vi "escape json string.vi"(11 "base string":string) -> (3 "String out":string)   [LabVIEW 2013, in "json generator.lvlib"]
uses:
  json generator.lvlib
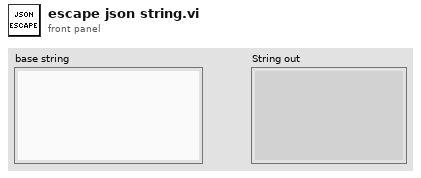
[diagram p1: front panel]
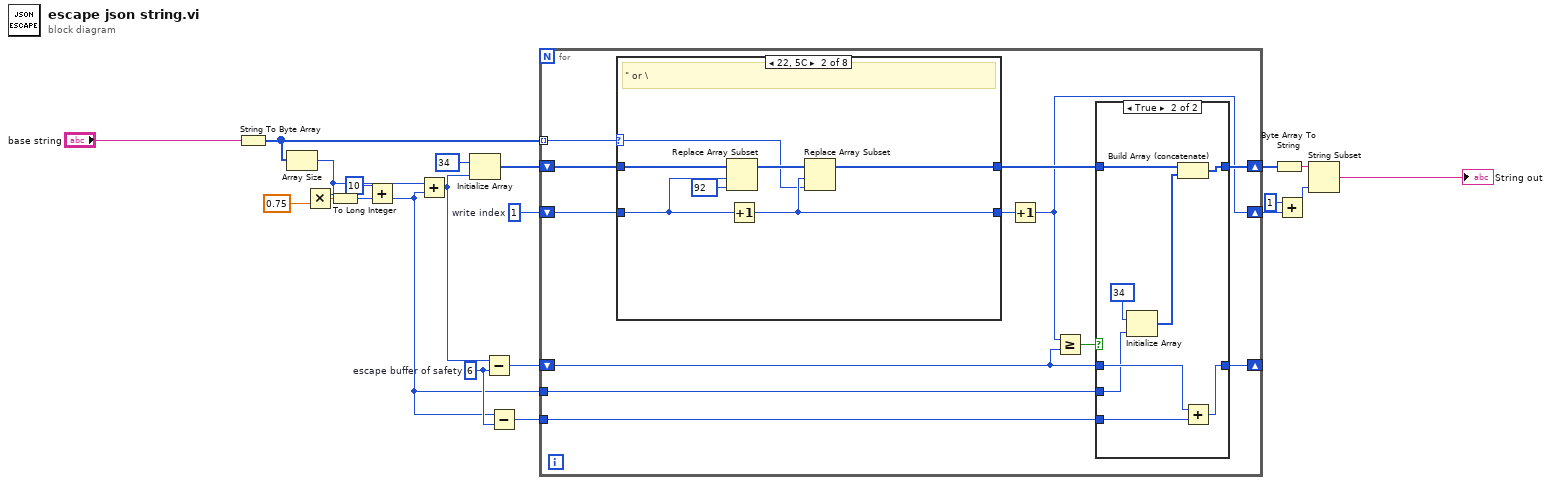
[diagram p0: block diagram]
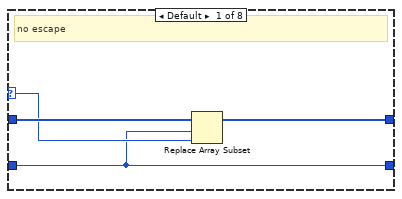
[diagram p3: hidden frame]
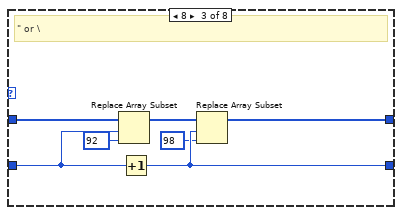
[diagram p4: hidden frame]
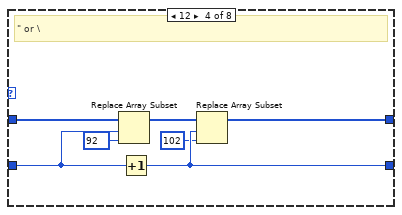
[diagram p5: hidden frame]
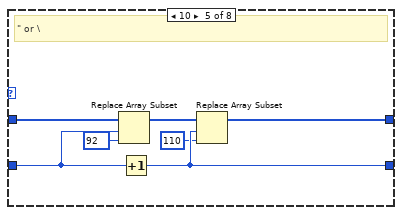
[diagram p6: hidden frame]
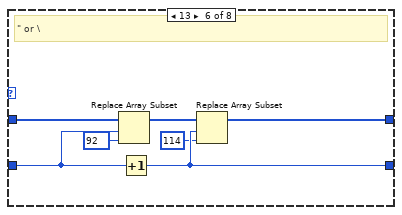
[diagram p7: hidden frame]
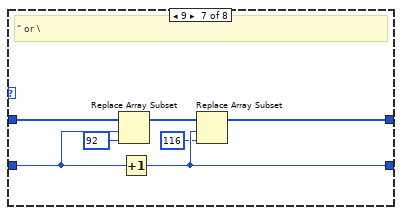
[diagram p8: hidden frame]
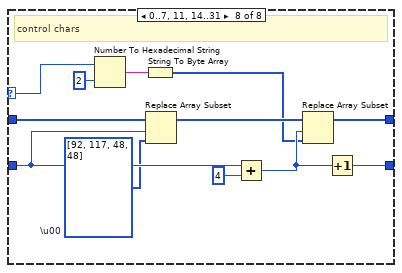
[diagram p9: hidden frame]
diagram:
  w6 = 6  # escape buffer of safety
  w18 = 1  # write index
  n1 = String To Byte Array(string="base string") -> (unsigned byte array=w12:u8[])
  n2 = Array Size(array=w12) -> (size(s)=w10:i32)
  n3 = Multiply(x=w10, y=0.75) -> (x*y=w13:dbl)
  n4 = To Long Integer(number=w13) -> (32bit integer=w7:i32)
  n5 = Add(x=10, y=w7) -> (x+y=w3:i32)
  n6 = Add(x=w10, y=w3) -> (x+y=w9:i32)
  n7 = Initialize Array(u8 34, w9) -> (w15:u8[])
  n8 = Subtract(x=w9, y=w6) -> (x-y=w8:i32)
  n9 = Subtract(x=w3, y=w6) -> (x-y=w5:i32)
  n10 = for {
    shift-right: [w30] -> w17
    shift-left: w15 -> [w33]
    shift-right: [w23] -> w11
    shift-left: w18 -> [w32]
    tunnel: w12 -> [w31] mode=indexing
    shift-right: [w27] -> _
    shift-left: w8 -> [w26]
    tunnel: w3 -> [w25]
    tunnel: w5 -> [w24]
    n11 = case shown="22, 5C" w31 {
      selector: w31 -> [w45 w49 _ _ _ _ _ w98]
      tunnel: w33 -> [w47 w54 w61 w68 w75 w82 w89 w101]
      tunnel: [w46 w51 w58 w65 w72 w79 w86 w100] -> w29
      tunnel: w32 -> [w44 w52 w59 w66 w73 w80 w87 w99]
      tunnel: [w44 w50 w57 w64 w71 w78 w85 w90] -> w28
      frame Default {
        # "no escape"
        n12 = Replace Array Subset(array=w47, new element=w45, index=w44) -> (w46:u8[])
      }
      frame 34, 92 {
        # "\" or \\"
        n13 = Replace Array Subset(array=w54, new element=u8 92 ("new element/subarray"), index=w52) -> (w53:u8[])
        n14 = Increment(x=w52) -> (x+1=w50:i32)
        n15 = Replace Array Subset(array=w53, new element=w49, index=w50) -> (w51:u8[])
      }
      frame 8 {
        # "\" or \\"
        n16 = Replace Array Subset(array=w61, new element=u8 92 ("new element/subarray"), index=w59) -> (w60:u8[])
        n17 = Increment(x=w59) -> (x+1=w57:i32)
        n18 = Replace Array Subset(array=w60, new element=u8 98 ("new element/subarray"), index=w57) -> (w58:u8[])
      }
      frame 12 {
        # "\" or \\"
        n19 = Replace Array Subset(array=w68, new element=u8 92 ("new element/subarray"), index=w66) -> (w67:u8[])
        n20 = Increment(x=w66) -> (x+1=w64:i32)
        n21 = Replace Array Subset(array=w67, new element=u8 102 ("new element/subarray"), index=w64) -> (w65:u8[])
      }
      frame 10 {
        # "\" or \\"
        n22 = Replace Array Subset(array=w75, new element=u8 92 ("new element/subarray"), index=w73) -> (w74:u8[])
        n23 = Increment(x=w73) -> (x+1=w71:i32)
        n24 = Replace Array Subset(array=w74, new element=u8 110 ("new element/subarray"), index=w71) -> (w72:u8[])
      }
      frame 13 {
        # "\" or \\"
        n25 = Replace Array Subset(array=w82, new element=u8 92 ("new element/subarray"), index=w80) -> (w81:u8[])
        n26 = Increment(x=w80) -> (x+1=w78:i32)
        n27 = Replace Array Subset(array=w81, new element=u8 114 ("new element/subarray"), index=w78) -> (w79:u8[])
      }
      frame 9 {
        # "\" or \\"
        n28 = Replace Array Subset(array=w89, new element=u8 92 ("new element/subarray"), index=w87) -> (w88:u8[])
        n29 = Increment(x=w87) -> (x+1=w85:i32)
        n30 = Replace Array Subset(array=w88, new element=u8 116 ("new element/subarray"), index=w85) -> (w86:u8[])
      }
      frame 0..7, 11, 14..31 {
        w91 = u8[] [92, 117, 48, 48]  # \u00
        # "control chars"
        n31 = Number To Hexadecimal String(1:i16 2 ("width (-)"), 2:w98) -> (0:w93:string)
        n32 = String To Byte Array(string=w93) -> (unsigned byte array=w95:u8[])
        n33 = Replace Array Subset(array=w101, new element=w91, index=w99) -> (w97:u8[])
        n34 = Add(x=w99, y=4) -> (x+y=w96:i32)
        n35 = Replace Array Subset(array=w97, new element=w95, index=w96) -> (w100:u8[])
        n36 = Increment(x=w96) -> (x+1=w90:i32)
      }
    }
    n37 = Increment(x=w28) -> (x+1=w23:i32)
    n38 = Greater Or Equal?(x=w23, y=w26) -> (x >= y?=w22:bool)
    n39 = case shown="True" w22 {
      tunnel: [w35 w38] -> w30
      tunnel: w29 -> [w35 w39]
      tunnel: [w34 w41] -> w27
      tunnel: w26 -> [w34 w42]
      tunnel: w25 -> [_ w40]
      tunnel: w24 -> [_ w43]
      frame False {
      }
      frame True {
        n40 = Initialize Array(u8 34, w40) -> (w37:u8[])
        n41 = Build Array (concatenate)(w39, w37) -> (w38:u8[])
        n42 = Add(x=w42, y=w43) -> (x+y=w41:i32)
      }
    }
  }
  n43 = Byte Array To String(unsigned byte array=w17) -> (string=w19:string)
  n44 = Add(x=1, y=w11) -> (x+y=w4:i32)
  n45 = String Subset(string=w19, length (rest)=w4) -> (substring=→"String out":string)  [unwired: 1 in]
